vi "Gas Set Setpoint SI.vi"(4 "Gas Set (0)":i32, 7 "Set? (F:Read)":bool, 8 "Error In":errorcluster, 9 "Flow Setpoint (0 l/min)":dbl[unit], 10 "Channel (0)":i32, 11 "VISA resource name":refnum<visa-resource-name>) -> (0 "Error Out":errorcluster, 1 "Flow Setpoint out":dbl[unit], 3 "dup VISA resource name":refnum<visa-resource-name>)   [LabVIEW 2011, in "MGC647C.lvlib"]
doc: "Read/Set flow setpoint of a channel in SI unit."
uses:
  <instrlib>/MGC647C/MGC647C.lvlib
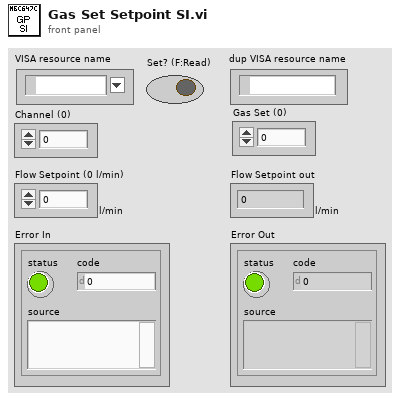
[diagram p1: front panel]
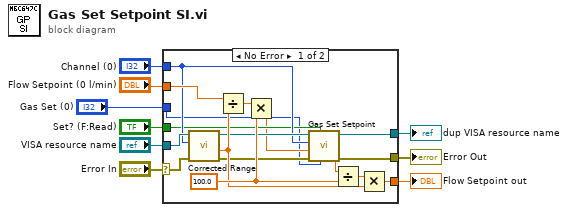
[diagram p0: block diagram]
diagram:
  n1 = case shown="No Error" "Error In" {
    selector: "Error In" -> [w19 w28]
    tunnel: "VISA resource name" -> [w20 w27]
    tunnel: [w16 w27] -> w8
    tunnel: [w17 w28] -> w7
    tunnel: "Set? (F:Read)" -> [w13 _]
    tunnel: "Flow Setpoint (0 l/min)" -> [w23 w29]
    tunnel: [w25 w29] -> w3
    tunnel: "Channel (0)" -> [w14 _]
    tunnel: "Gas Set (0)" -> [w10 _]
    frame No Error {
      w22 = 100.0 ("y")
      n2 = call <instrlib>:"Corrected Range.vi"("Error In"=w19, "Channel (0)"=w14, "VISA resource name"=w20) -> ("Error Out"=w18:errorcluster, "Corrected Range"=w21:dbl[unit], "dup VISA resource name"=w15:refnum<visa-resource-name>)  [unwired: 6 in]
      n3 = Divide(x=w23, y=w21) -> (x/y=w24:dbl)
      n4 = Multiply(x=w24, y=w22) -> (x*y=w12:dbl)
      n5 = call <instrlib>:"Gas Set Setpoint.vi"("Gas Set (0)"=w10, "Set? (F:Read)"=w13, "Error In"=w18, "Setpoint (0%)"=w12, "Channel (0)"=w14, "VISA resource name"=w15) -> ("Error Out"=w17:errorcluster, "Setpoint out"=w11:dbl, "dup VISA resource name"=w16:refnum<visa-resource-name>)  [unwired: 3 in]
      n6 = Divide(x=w11, y=w22) -> (x/y=w26:dbl)
      n7 = Multiply(x=w26, y=w21) -> (x*y=w25:dbl[unit])
    }
    frame Error {
    }
  }
  "dup VISA resource name" <- w8
  "Error Out" <- w7
  "Flow Setpoint out" <- w3
